vi "BRig_RT__Case_Exp__recordAnalogInput__PortC__netstream_noBuffer.vi"(0 "input_countTO":u32, 2 "input_iOccurence":u16, 3 "resetOccurrence":bool, 4 "input_dataCurrent":u16[](array[numeric]), 5 "input_empytyArray":u16[](array[numeric]), 6 "input_iState_start":T1, 7 "input_fifo_hdl":refnum<k33>, 8 "input_iState_end":T1, 9 "input_fifo_error":errorcluster, 10 "input_AI1":i16, 12 "input_AI0":i16) -> (11 "output_fifo_hdl":refnum<k33>, 13 "error out":errorcluster, 14 "output_countTO":u32, 16 "output_iOccurrence":u16)   [LabVIEW 2014]
uses:
  myRIO_BRig_RT__Case_Exp_stateList.ctl
panel:
  out "error out 2":errorcluster
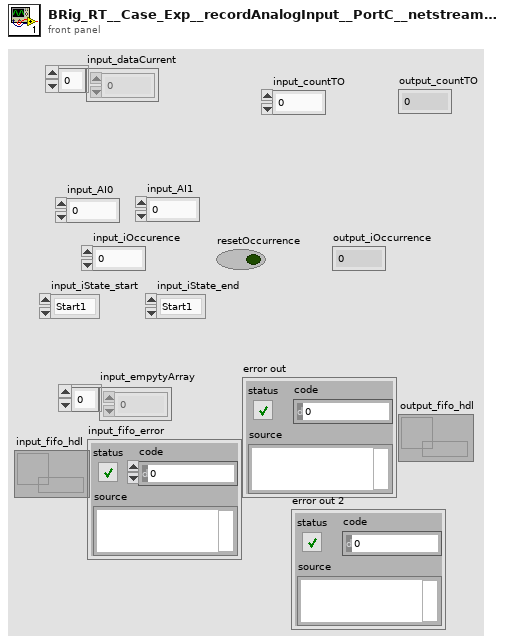
[diagram p1: front panel]
types:
  T1 = typedef "myRIO_BRig_RT__Case_Exp_stateList.ctl" = enum16{"Start1", "Start2", "Start3", "saveSettings1", "saveSettings2", "saveSettings3", "saveSettings4", "saveSettings_LC_ENL_l1", "saveSettings_LC_ENL_l2", "saveSettings_LC_Cue_l1", "saveSettings_LC_Cue_l2", "saveSettings6_LC_l1_Other", "SaveSettings6_LC_l2_Other", "setSettings_Audio", "setSettings_Laser", "initBlock_pre", "initBlock", "initBlock2", "initBlock_post", "initTrial_pre", "initTrial", "initTrial2", "initTrial3", "initTrial4", "initTrial_LC_ENL1", "initTrial_LC_Cue1", "initTrial_LC_Cue1_2", "initTrial_LC_Sel", "initTrial_post", "ENL1_pre", "ENL1", "ENL1_post", "ENL1Penalty_pre", "ENL1Penalty", "ENL2_pre", "ENL2", "ENL2Penalty_pre", "ENL2Penalty", "Cue1_pre", "Cue1", "Cue1_post", "Cue1Penalty_pre", "Cue1Penalty", "Cue2_pre", "Cue2", "Cue2Penalty_pre", "Cue2Penalty", "Selection_pre", "Selection", "Select_post", "SelectReward_pre", "SelectReward", "SelectRewardPost_pre", "SelectRewardPost", "SelectWrong_pre", "SelectWrong", "SelectWrong_post", "SelectTimeout_pre", "SelectTimeout", "SelectTimeout_post", "endTrial_pre", "endTrial1", "endTrial2", "endTrial3", "endTrial_post", "endBlock_pre", "endBlock", "endBlock_post", "endExp", "commConnect", "commUpload_pre", "commUpload_dataBlock", "commUpload_dataCurrent", "commUpload_dataExp", "commUpload_dataLC", "commUpload_dataTrial", "commUpload_post", "saveData_pre", "saveData_dataBlock", "saveData_dataCurrent", "saveData_dataExp", "saveData_dataLC", "saveData_dataTrial", "saveData_post", "empty_endBlock1", "empty_endBlock2", "empty_endTrial1", "empty_endTrial2", "empty_endTrial3", "empty_endTrial4", "empty_endTrial5", "dummyState", "dummyState_endBlock", "FreeReward_pre", "FreeReward", "FreeRewardPost_pre", "FreeRewardPost"}
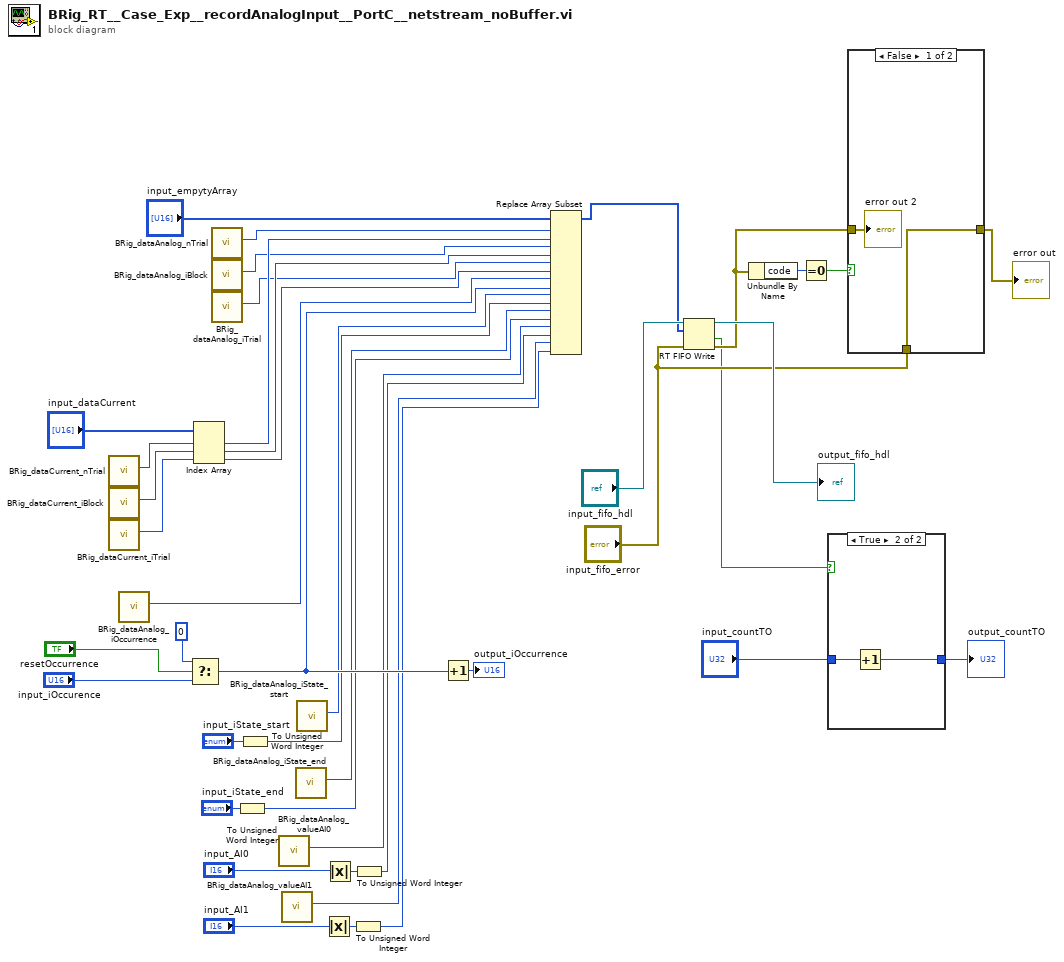
[diagram p0: block diagram]
diagram:
  n1 = call "BRig_dataCurrent_nTrial.vi"() -> ("output_nTrial"=w39:i32)  [unwired: 11 in]
  n2 = call "BRig_dataCurrent_iBlock.vi"() -> ("output_iBlock"=w38:i32)  [unwired: 11 in]
  n3 = call "BRig_dataCurrent_iTrial.vi"() -> ("output_iTrial"=w37:i32)  [unwired: 11 in]
  n4 = call "BRig_dataAnalog_iOccurrence.vi"() -> ("output_iOccurrence"=w20:i32)  [unwired: 11 in]
  n5 = Select(t=u16 0, s="resetOccurrence", f="input_iOccurence") -> (s? t:f=w19:u16)
  n6 = Index Array(array="input_dataCurrent", index #1=w39, index #2=w38, index #3=w37) -> (element #1=w25:u16, element #2=w23:u16, element #3=w21:u16)
  n7 = call "BRig_dataAnalog_nTrial.vi"() -> ("output_nTrial"=w26:i32)  [unwired: 11 in]
  n8 = call "BRig_dataAnalog_iBlock.vi"() -> ("output_iBlock"=w24:i32)  [unwired: 11 in]
  n9 = call "BRig_dataAnalog_iTrial.vi"() -> ("output_iTrial"=w22:i32)  [unwired: 11 in]
  n10 = To Unsigned Word Integer(number="input_iState_end") -> (unsigned 16bit integer=w15:u16)
  n11 = To Unsigned Word Integer(number="input_iState_start") -> (unsigned 16bit integer=w17:u16)
  n12 = call "BRig_dataAnalog_valueAI0.vi"() -> ("output_valueAI0"=w14:i32)  [unwired: 11 in]
  n13 = call "BRig_dataAnalog_valueAI1.vi"() -> ("output_valueAI1"=w12:i32)  [unwired: 11 in]
  n14 = call "BRig_dataAnalog_iState_end.vi"() -> ("output_iState_end"=w16:i32)  [unwired: 11 in]
  n15 = call "BRig_dataAnalog_iState_start.vi"() -> ("output_iState_start"=w18:i32)  [unwired: 11 in]
  n16 = Absolute Value(x="input_AI1") -> (abs(x)=w41:i16)
  n17 = Absolute Value(x="input_AI0") -> (abs(x)=w42:i16)
  n18 = To Unsigned Word Integer(number=w41) -> (unsigned 16bit integer=w11:u16)
  n19 = To Unsigned Word Integer(number=w42) -> (unsigned 16bit integer=w13:u16)
  n20 = Increment(x=w19) -> (x+1=→"output_iOccurrence":u16)
  n21 = Replace Array Subset(array="input_empytyArray", new element #1=w25, index #1=w26, new element #2=w23, index #2=w24, new element #3=w21, index #3=w22, new element #4=w19, index #4=w20, new element #5=w17, index #5=w18, new element #6=w15, index #6=w16, new element #7=w13, index #7=w14, new element #8=w11, index #8=w12) -> (w7:u16[])
  n22 = RT FIFO Write(0:"input_fifo_hdl", 1:w7, 3:"input_fifo_error") -> (8:→"output_fifo_hdl":refnum<k33>, 10:w3:bool, 11:w5:errorcluster)  [unwired: 2 in, 1 out]
  n23 = Unbundle By Name(w5) -> ("code"=w28:i32)
  n24 = Equal To 0?(x=w28) -> (x = 0?=w10:bool)
  n25 = case shown="True" w3 {
    tunnel: "input_countTO" -> [w43 w45]
    tunnel: [w43 w44] -> w1
    frame False {
    }
    frame True {
      n26 = Increment(x=w45) -> (x+1=w44:u32)
    }
  }
  "output_countTO" <- w1
  n27 = case shown="False" w10 {
    tunnel: w5 -> [w46 w48]
    tunnel: [w47 w48] -> w9
    tunnel: "input_fifo_error" -> [w47 _]
    frame False {
      "error out 2" <- w46
    }
    frame True {
    }
  }
  "error out" <- w9
